vi "Dispose.vi"(8 "error in (no error)":errorcluster, 11 "Wall":refnum<class "Wall.lvclass">) -> (0 "error out":errorcluster)   [LabVIEW 2020, in "Wall.lvclass"]
uses:
  Wall.lvclass
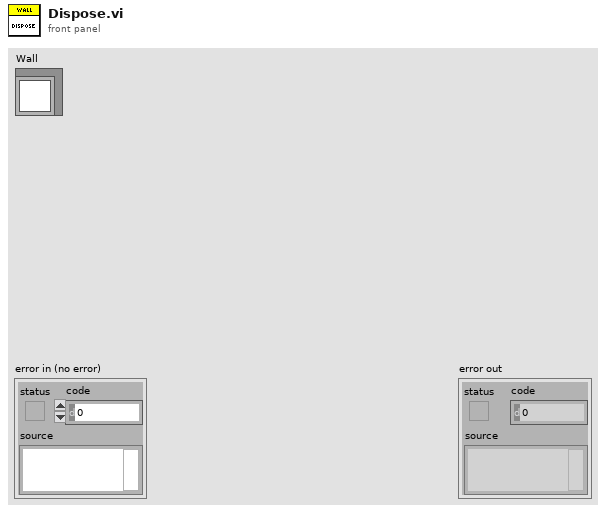
[diagram p1: front panel]
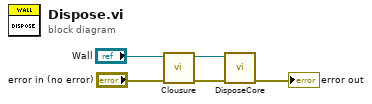
[diagram p0: block diagram]
diagram:
  n1 = call-dynamic "Clousure.vi"("error in (no error)"="error in (no error)", "Wall"="Wall") -> ("error out"=w3:errorcluster, "Wall"=w4:refnum<class "Wall.lvclass">)  [unwired: 8 in]
  n2 = call-dynamic "DisposeCore.vi"("error in (no error)"=w3, "Wall"=w4) -> ("error out"=→"error out":errorcluster)  [unwired: 8 in, 1 out]
